vi "main.vi"() -> ()   [LabVIEW 2018]
doc: "This example demonstrates the use of binary morphological reconstruction in the particle analysis. The example allows you to keep the particles completely inside the ROI, completely outside the ROI or on the ROI."
uses:
  <vilib>/vision/NI_Vision_Development_Module.lvlib
panel:
  in  "Font, Size & Style":T1={"Desired Font (Application)"=enum."Application Font", "[User-specified Font]"={"Font Name"="", "Size"=12, "Strikeout?"=FALSE, "Italic?"=FALSE, "Underline?"=FALSE, "Outline?"=FALSE, "Shadow?"=FALSE, "Bold?"=FALSE, "Rotation Angle"=0.0}, "Horizontal Alignment"=0, "Vertical Alignment"=0} {"Horizontal Alignment" items=["Left", "Center", "Right"]; "Vertical Alignment" items=["Bottom", "Top", "Baseline"]}
  in  "Font, Size & Style 3":T1={"Desired Font (Application)"=enum."Application Font", "[User-specified Font]"={"Font Name"="", "Size"=12, "Strikeout?"=FALSE, "Italic?"=FALSE, "Underline?"=FALSE, "Outline?"=FALSE, "Shadow?"=FALSE, "Bold?"=FALSE, "Rotation Angle"=0.0}, "Horizontal Alignment"=0, "Vertical Alignment"=0} {"Vertical Alignment" items=["Bottom", "Top", "Baseline"]; "Horizontal Alignment" items=["Left", "Center", "Right"]; "[User-specified Font]"."Rotation Angle" format="%.2f"}
  out "总面积":i32
  out "ROI左上角坐标":cluster{i32, i32}
  out "透射图灰度表":u32[](graph)
  out "全图灰度级信息":T2 {"标准差" format="%.2f"; "均值" format="%.2f"; "相邻灰度级间隔" format="%.2f"; "起始灰度值" format="%.2f"; "最大值" format="%.2f"; "最小值" format="%.2f"}
  out "最大灰度值":sgl
  out "标注图":T3(plugin-control)
  out "写入数据库路径":path
  out "反射图灰度表":u32[](graph)
  out "反射图":T3(plugin-control)
  out "最大灰度值":sgl
  out "框数":dbl
  out "全图灰度级信息":T2 {"标准差" format="%.2f"; "均值" format="%.2f"; "相邻灰度级间隔" format="%.2f"; "起始灰度值" format="%.2f"; "最大值" format="%.2f"; "最小值" format="%.2f"}
  in  "评定报告生成":bool
  in  "部位":string
  in  "产品序号":string
  in  "测试人":string
  in  "预处理":bool
  in  "查看标注":bool
  in  "导入图像":bool
  in  "删除标注":bool
  in  "退出":bool
  in  "Font, Size & Style 2":T1={"Desired Font (Application)"=enum."Application Font", "[User-specified Font]"={"Font Name"="", "Size"=12, "Strikeout?"=FALSE, "Italic?"=FALSE, "Underline?"=FALSE, "Outline?"=FALSE, "Shadow?"=FALSE, "Bold?"=FALSE, "Rotation Angle"=0.0}, "Horizontal Alignment"=0, "Vertical Alignment"=0} {"Vertical Alignment" items=["Bottom", "Top", "Baseline"]; "Horizontal Alignment" items=["Left", "Center", "Right"]; "[User-specified Font]"."Rotation Angle" format="%.2f"}
  out "框组":T4(array[cluster])
  in  "Operation":enum16{"overlay rectangle"}(ring)
  # "穿透法图像"
  # "反射法图像"
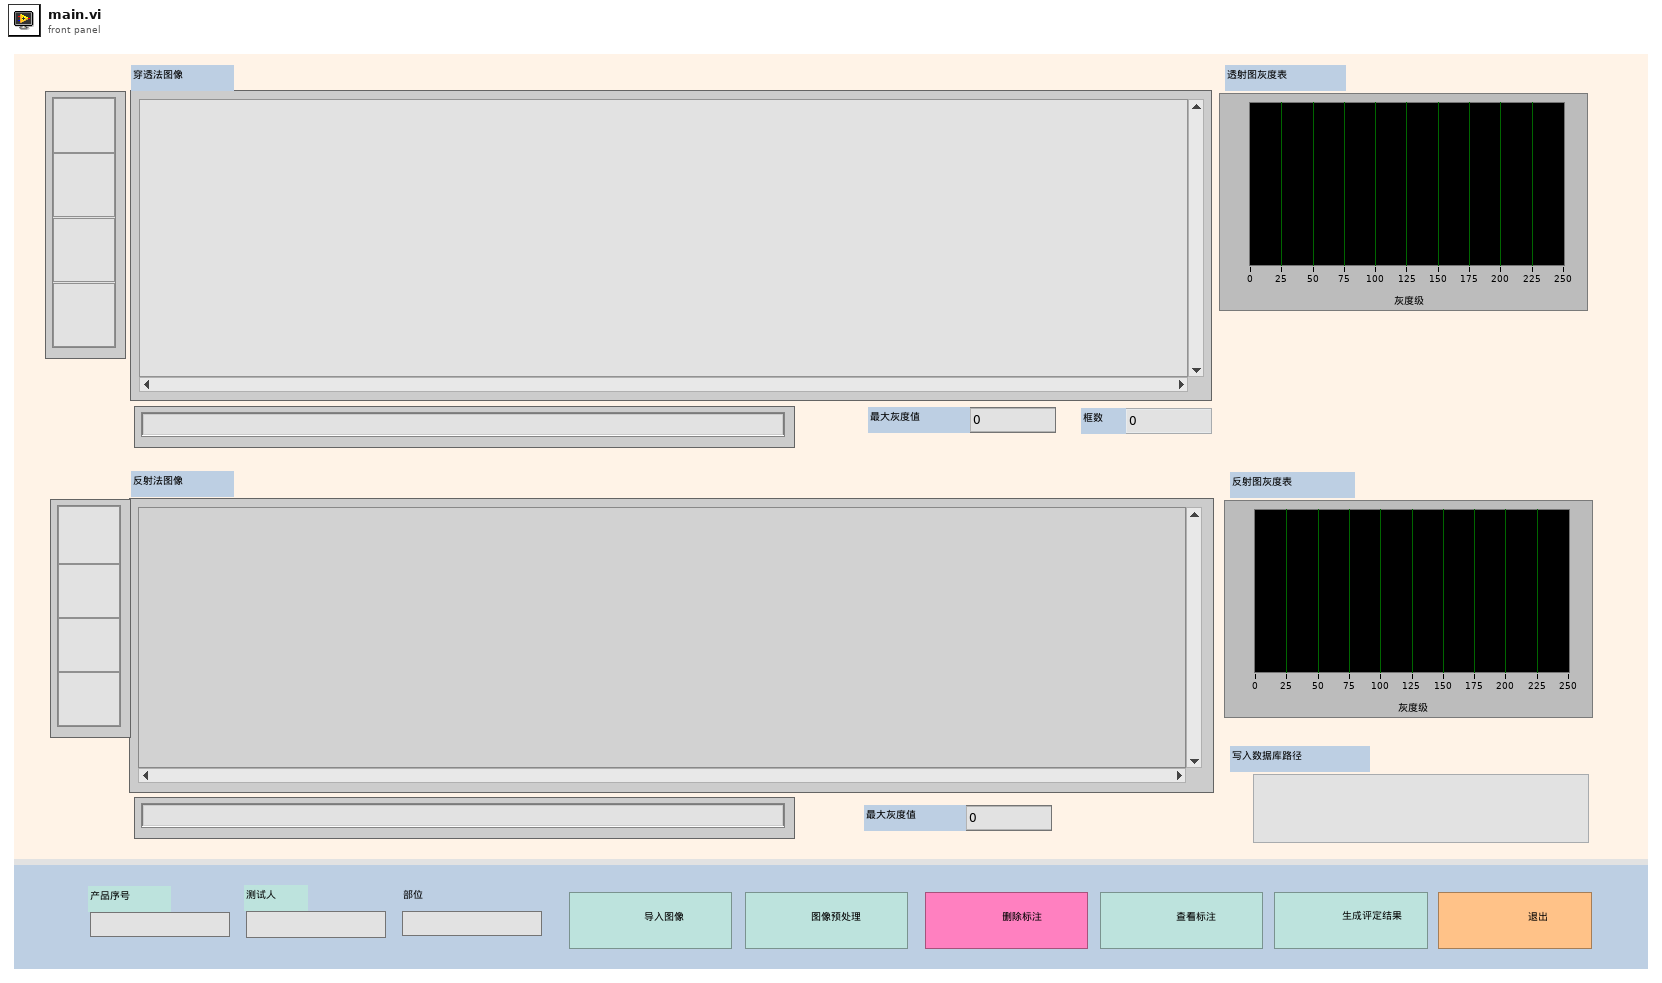
[diagram p1: front panel]
types:
  T1 = cluster{"Desired Font (Application)":enum16{"User-specified Font", "Application Font", "System Font", "Dialog Font"}, "[User-specified Font]":cluster{"Font Name":string, "Size":i16, "Strikeout?":bool, "Italic?":bool, "Underline?":bool, "Outline?":bool, "Shadow?":bool, "Bold?":bool, "Rotation Angle":dbl}, "Horizontal Alignment":i16, "Vertical Alignment":i16}
  T2 = cluster{"histogram":u32[], "最小值":sgl, "最大值":sgl, "起始灰度值":sgl, "相邻灰度级间隔":sgl, "均值":sgl, "标准差":sgl, "像素面积":i32}
  T3 = typedef "IMAQ Image.ctl" = refnum<image>
  T4 = cluster{"Global Rectangle":i32[], "Contours":cluster{"Contour Type":u32, "ROI Type":u32, "Points":i32[]}[]}[]
  T5 = typedef "Image Type" = u32
  T6 = cluster{"Global Rectangle":i32[], "Contours":cluster{"Contour Type":u32, "ROI Type":u32, "Points":i32[]}[]}
  T7 = cluster{"histogram":u32[], "Minimal Value":sgl, "Maximal Value":sgl, "Starting Value":sgl, "Interval Width":sgl, "Mean Value":sgl, "Standard  Variation":sgl, "Area (pixels)":i32}
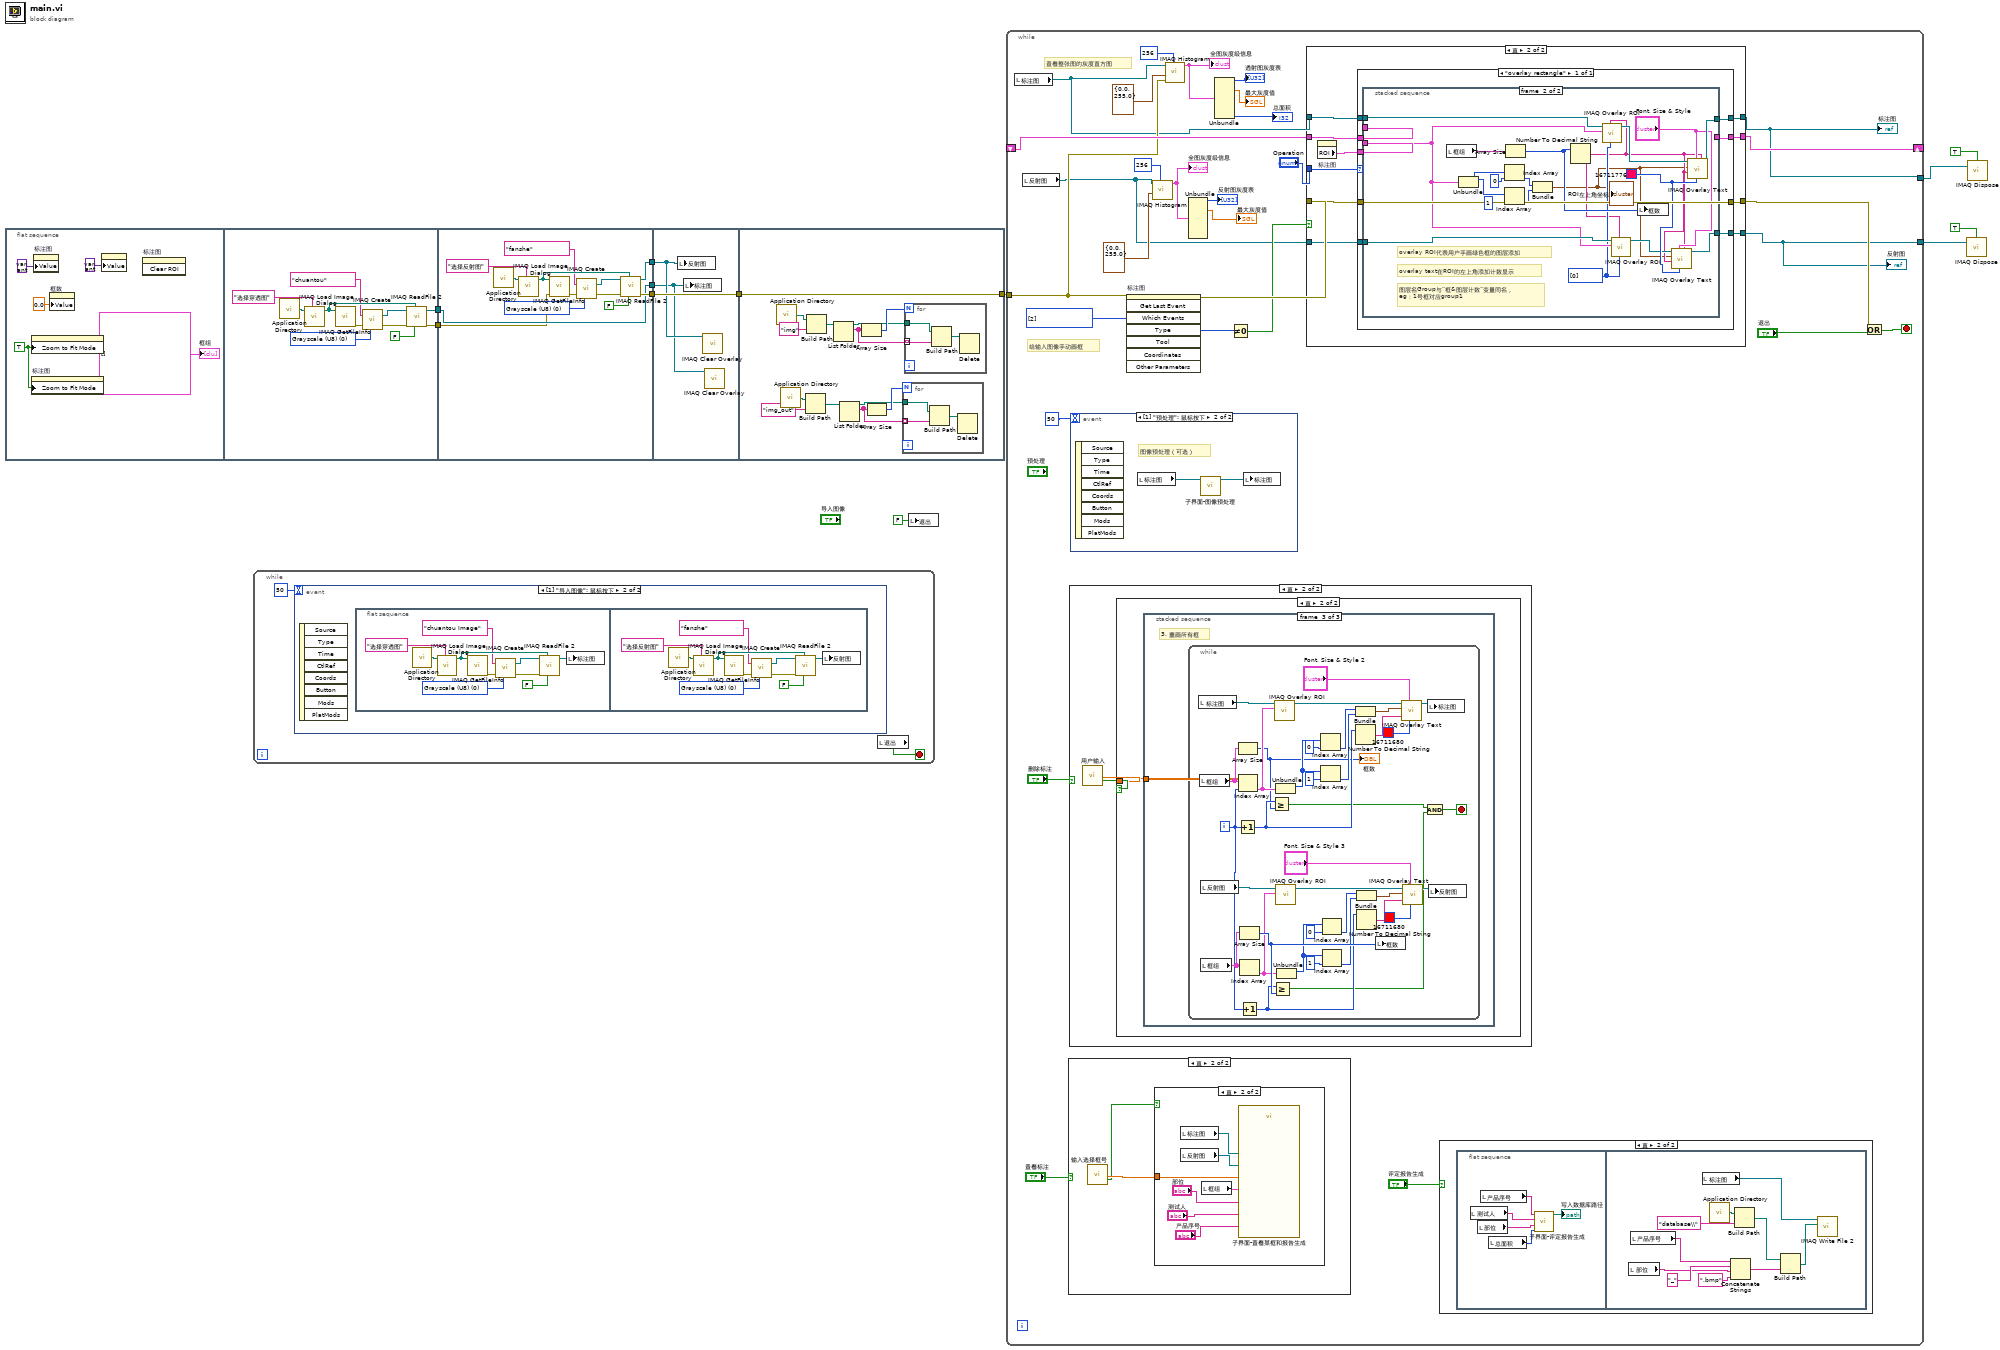
[diagram p0: block diagram]
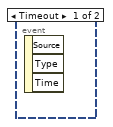
[diagram p2: hidden frame]
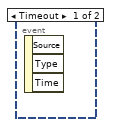
[diagram p4: hidden frame]
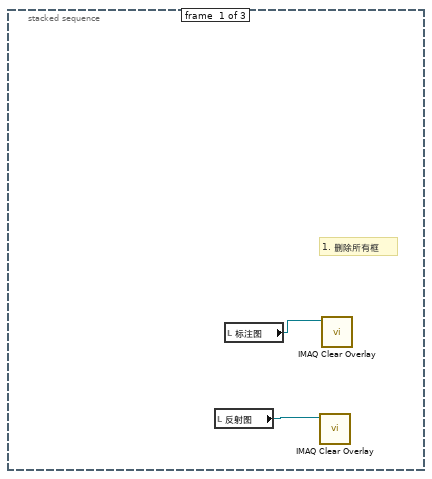
[diagram p9: hidden frame]
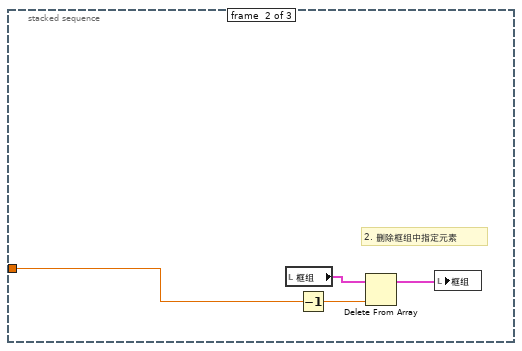
[diagram p10: hidden frame]
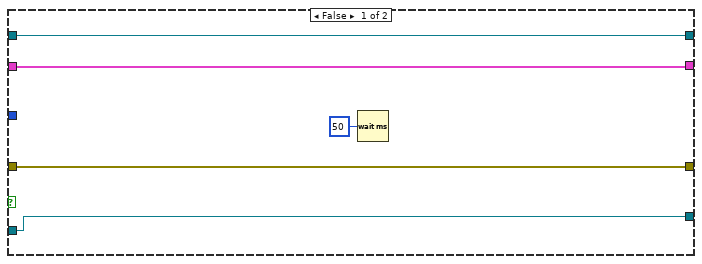
[diagram p11: hidden frame]
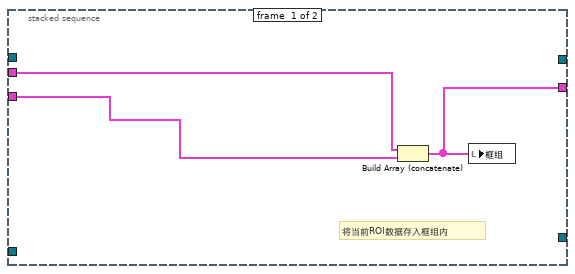
[diagram p12: hidden frame]
diagram:
  n1 = flat-sequence {
    tunnel: [w19] -> w9
    tunnel: [w18] -> w8
    tunnel: w9 -> [w30]
    tunnel: w8 -> [w31]
    tunnel: [w32] -> w7
    tunnel: [w31] -> w6
    tunnel: [w29] -> w5
    tunnel: w7 -> [w44]
    tunnel: w6 -> [w42]
    tunnel: w5 -> [w43]
    tunnel: [w44] -> w1
    tunnel: [w57] -> w12
    tunnel: w1 -> [w57]
    frame #0 {
      w16 = TRUE ("Zoom to Fit Mode")
      n2 = property on="反射图" class="ImageControl"("Zoom to Fit Mode"=w16) -> ()  [unwired: 2 in, 2 out]
      n3 = property on="标注图" class="ImageControl"("Zoom to Fit Mode"=w16) -> ()  [unwired: 2 in, 2 out]
      n4 = property on="标注图" class="ImageControl"("Value"=variant ("值")) -> ()  [unwired: 2 in, 2 out]
      n5 = property on="框数" class="DigNum (严格)"("Value"=0.0 ("标注框总数")) -> ()  [unwired: 2 in, 2 out]
      n6 = property on="反射图" class="ImageControl"("Value"=variant ("值")) -> ()  [unwired: 2 in, 2 out]
      n7 = invoke on="标注图" class="ImageControl" method="Clear ROI"() -> ()  [unwired: 3 in, 3 out]
      "框组" <- T4 [] ("框组")
    }
    frame #1 {
      w20 = T5 0 items=["Grayscale (U8)", "Grayscale (I16)", "Grayscale (SGL)", "Complex (CSG)", "RGB (U32)", "HSL (U32)", "RGB (U64)", "Grayscale (U16)"] ("Image Type")
      n8 = call <vilib>:"Application Directory.vi"() -> ("Application Directory"=w28:path)
      n9 = call "IMAQ Load Image Dialog"("Prompt"="选择穿透图" ("prompt"), "Start Path"=w28) -> ("Path"=w24:path)  [unwired: 7 in, 2 out]
      n10 = call "IMAQ GetFileInfo"("File Path"=w24) -> ("error out"=w25:errorcluster)  [unwired: 4 in, 6 out]
      n11 = call "IMAQ Create"("Image Name"="chuantou", "Image Type"=w20, "error in (no error)"=w25) -> ("New Image"=w26:T3, "error out"=w27:errorcluster)  [unwired: 2 in]
      n12 = call "IMAQ ReadFile 2"("Use File Path Image Type"=FALSE, "File Path"=w24, "error in (no error)"=w27, "Image"=w26) -> ("error out"=w19:errorcluster, "Image Out"=w18:T3)  [unwired: 3 in, 3 out]
    }
    frame #2 {
      w33 = T5 0 items=["Grayscale (U8)", "Grayscale (I16)", "Grayscale (SGL)", "Complex (CSG)", "RGB (U32)", "HSL (U32)", "RGB (U64)", "Grayscale (U16)"] ("Image Type")
      n13 = call <vilib>:"Application Directory.vi"() -> ("Application Directory"=w41:path)
      n14 = call "IMAQ Load Image Dialog"("Prompt"="选择反射图" ("prompt"), "Start Path"=w41) -> ("Path"=w37:path)  [unwired: 7 in, 2 out]
      n15 = call "IMAQ GetFileInfo"("error in (no error)"=w30, "File Path"=w37) -> ("error out"=w38:errorcluster)  [unwired: 3 in, 6 out]
      n16 = call "IMAQ Create"("Image Name"="fanshe", "Image Type"=w33, "error in (no error)"=w38) -> ("New Image"=w39:T3, "error out"=w40:errorcluster)  [unwired: 2 in]
      n17 = call "IMAQ ReadFile 2"("Use File Path Image Type"=FALSE, "File Path"=w37, "error in (no error)"=w40, "Image"=w39) -> ("error out"=w32:errorcluster, "Image Out"=w29:T3)  [unwired: 3 in, 3 out]
    }
    frame #3 {
      n18 = local write "反射图"(w43) -> ()
      n19 = local write "标注图"(w42) -> ()
      n20 = call "IMAQ Clear Overlay"("Image"=w43) -> ()  [unwired: 9 in, 2 out]
      n21 = call "IMAQ Clear Overlay"("Image"=w42) -> ()  [unwired: 9 in, 2 out]
    }
    frame #4 {
      n22 = call <vilib>:"Application Directory.vi"() -> ("Application Directory"=w53:path)
      n23 = call <vilib>:"Application Directory.vi"() -> ("Application Directory"=w47:path)
      n24 = Build Path(base path=w47, name or relative path="img_out" ("名称或相对路径")) -> (appended path=w48:path)
      n25 = Build Path(base path=w53, name or relative path="img" ("名称或相对路径")) -> (appended path=w54:path)
      n26 = List Folder(path=w54) -> (path out=w52:path, filenames=w56:string[])  [unwired: 3 in, 2 out]
      n27 = List Folder(path=w48) -> (path out=w46:path, filenames=w50:string[])  [unwired: 3 in, 2 out]
      n28 = Array Size(array=w56) -> (size(s)=w55:i32)
      n29 = Array Size(array=w50) -> (size(s)=w49:i32)
      n30 = for {
        N: w49 -> [_]
        tunnel: w46 -> [w59]
        tunnel: w50 -> [w58] mode=indexing
        n31 = Build Path(base path=w59, name or relative path=w58) -> (appended path=w60:path)
        n32 = Delete(path (use dialog)=w60) -> ()  [unwired: 4 in, 3 out]
      }
      n33 = for {
        N: w55 -> [_]
        tunnel: w52 -> [w62]
        tunnel: w56 -> [w61] mode=indexing
        n34 = Build Path(base path=w62, name or relative path=w61) -> (appended path=w63:path)
        n35 = Delete(path (use dialog)=w63) -> ()  [unwired: 4 in, 3 out]
      }
    }
  }
  n36 = while {
    stop <- w64 stop-if-true
    n37 = event shown="[1] \"导入图像\": 鼠标按下" {
      selector: _ -> [_ _]
      dyn-events: _ -> [_ _]
      timeout: 50 -> [_ _]
      event Timeout {
        n38 = event-data() -> ()  [unwired: 1 in, 3 out]
      }
      event "导入图像": Mouse Down {
        n39 = event-data() -> ()  [unwired: 1 in, 8 out]
        n40 = flat-sequence {
          frame #0 {
            w67 = T5 0 items=["Grayscale (U8)", "Grayscale (I16)", "Grayscale (SGL)", "Complex (CSG)", "RGB (U32)", "HSL (U32)", "RGB (U64)", "Grayscale (U16)"] ("Image Type")
            n41 = call <vilib>:"Application Directory.vi"() -> ("Application Directory"=w75:path)
            n42 = call "IMAQ Load Image Dialog"("Prompt"="选择穿透图" ("prompt"), "Start Path"=w75) -> ("Path"=w71:path)  [unwired: 7 in, 2 out]
            n43 = call "IMAQ GetFileInfo"("File Path"=w71) -> ("error out"=w72:errorcluster)  [unwired: 4 in, 6 out]
            n44 = call "IMAQ Create"("Image Name"="chuantou Image", "Image Type"=w67, "error in (no error)"=w72) -> ("New Image"=w73:T3, "error out"=w74:errorcluster)  [unwired: 2 in]
            n45 = call "IMAQ ReadFile 2"("Use File Path Image Type"=FALSE, "File Path"=w71, "error in (no error)"=w74, "Image"=w73) -> ("Image Out"=w66:T3)  [unwired: 3 in, 4 out]
            n46 = local write "标注图"(w66) -> ()
          }
          frame #1 {
            w79 = T5 0 items=["Grayscale (U8)", "Grayscale (I16)", "Grayscale (SGL)", "Complex (CSG)", "RGB (U32)", "HSL (U32)", "RGB (U64)", "Grayscale (U16)"] ("Image Type")
            n47 = call <vilib>:"Application Directory.vi"() -> ("Application Directory"=w81:path)
            n48 = call "IMAQ Load Image Dialog"("Prompt"="选择反射图" ("prompt"), "Start Path"=w81) -> ("Path"=w85:path)  [unwired: 7 in, 2 out]
            n49 = call "IMAQ GetFileInfo"("File Path"=w85) -> ("error out"=w84:errorcluster)  [unwired: 4 in, 6 out]
            n50 = call "IMAQ Create"("Image Name"="fanshe", "Image Type"=w79, "error in (no error)"=w84) -> ("New Image"=w83:T3, "error out"=w82:errorcluster)  [unwired: 2 in]
            n51 = call "IMAQ ReadFile 2"("Use File Path Image Type"=FALSE, "File Path"=w85, "error in (no error)"=w82, "Image"=w83) -> ("Image Out"=w76:T3)  [unwired: 3 in, 4 out]
            n52 = local write "反射图"(w76) -> ()
          }
        }
      }
    }
    n53 = local read "退出"() -> (w64:bool)
  }
  n54 = local write "退出"(FALSE ("退出")) -> ()
  n55 = while {
    shift-right: [w108] -> _
    shift-left: _ -> [w107]
    tunnel: w12 -> [w106]
    tunnel: [w90] -> w10
    tunnel: [w91] -> w3
    stop <- w110 stop-if-true
    (unwired) "_" ("名称或相对路径")
    (unwired) ".docx" ("名称或相对路径")
    w113 = i32[] [2] items=["No Event"=0, "Click Event"=1, "Draw Event"=2, "Size Event"=4, "Scroll Event"=5, "Double Click Event"=8] ("Which Events")
    # "给输入图像手动画框"
    # "查看整张图的灰度直方图"
    n56 = local read "标注图"() -> (w92:T3)
    n57 = local read "反射图"() -> (w93:T3)
    n58 = case shown="真" "查看标注" {
      frame False {
      }
      frame True {
        n59 = call "输入选择框号"() -> ("框号"=w134:dbl, "确定"=w133:bool)  [unwired: 17 in, 1 out]
        n60 = case shown="真" w133 {
          tunnel: w134 -> [_ w141]
          frame False {
            # "用户取消操作"
          }
          frame True {
            n61 = local read "标注图"() -> (w138:T3)
            n62 = local read "反射图"() -> (w139:T3)
            n63 = local read "框组"() -> (w140:T4)
            n64 = call "子界面-查看某框和报告生成.vi"("测试人"="测试人", "标注图"=w138, "部位"="部位", "产品序号"="产品序号", "反射图"=w139, "框组"=w140, "框号"=w141) -> ()  [unwired: 3 in]
          }
        }
      }
    }
    n65 = case shown="真" "删除标注" {
      frame False {
      }
      frame True {
        n66 = call "用户输入"() -> ("框号"=w142:dbl, "确定"=w143:bool)  [unwired: 17 in, 1 out]
        n67 = case shown="真" w143 {
          tunnel: w142 -> [_ w144]
          frame False {
            # "用户取消操作"
          }
          frame True {
            n68 = stacked-sequence {
              tunnel: w144 -> [_ w149 _]
              frame #0 {
                # "1. 删除所有框"
                n69 = local read "反射图"() -> (w145:T3)
                n70 = local read "标注图"() -> (w146:T3)
                n71 = call "IMAQ Clear Overlay"("Image"=w145) -> ()  [unwired: 9 in, 2 out]
                n72 = call "IMAQ Clear Overlay"("Image"=w146) -> ()  [unwired: 9 in, 2 out]
              }
              frame #1 {
                # "2. 删除框组中指定元素"
                n73 = local read "框组"() -> (w150:T4)
                n74 = Decrement(x=w149) -> (x-1=w148:dbl)
                n75 = Delete From Array(array=w150, index=w148) -> (array with subset deleted=w147:T4)  [unwired: 1 in, 1 out]
                n76 = local write "框组"(w147) -> ()
              }
              frame #2 {
                # "3. 重画所有框"
                n77 = while {
                  i -> [w155]
                  stop <- w152 stop-if-true
                  n78 = local read "标注图"() -> (w186:T3)
                  n79 = local read "框组"() -> (w180:T4)
                  n80 = local read "反射图"() -> (w156:T3)
                  n81 = local read "框组"() -> (w162:T4)
                  n82 = Array Size(array=w180) -> (size(s)=w171:i32)
                  "框数" <- w171
                  n83 = Index Array(array=w180, index=w155) -> (element=w173:T6)
                  n84 = Increment(x=w155) -> (x+1=w185:i32)
                  n85 = Array Size(array=w162) -> (size(s)=w170:i32)
                  n86 = Index Array(array=w162) -> (element=w169:T6)  [unwired: 1 in]
                  n87 = Increment(x=w155) -> (x+1=w157:i32)
                  n88 = Greater Or Equal?(x=w185, y=w171) -> (x >= y?=w154:bool)
                  n89 = Greater Or Equal?(x=w157, y=w170) -> (x >= y?=w153:bool)
                  n90 = call "IMAQ Overlay ROI"("ROI Descriptor"=w173, "Image"=w186) -> ("Image Out"=w182:T3)  [unwired: 8 in, 1 out]
                  n91 = Unbundle(w173) -> ("Global Rectangle"=w176:i32[])  [unwired: 1 out]
                  n92 = call "IMAQ Overlay ROI"("ROI Descriptor"=w169, "Image"=w156) -> ("Image Out"=w160:T3)  [unwired: 8 in, 1 out]
                  n93 = Unbundle(w169) -> ("Global Rectangle"=w166:i32[])  [unwired: 1 out]
                  n94 = Index Array(array=w176, index=0 ("索引")) -> (element=w177:i32)
                  n95 = Index Array(array=w176, index=1 ("索引")) -> (element=w178:i32)
                  n96 = Index Array(array=w166, index=0 ("索引")) -> (element=w165:i32)
                  n97 = Index Array(array=w166, index=1 ("索引")) -> (element=w164:i32)
                  n98 = Bundle(w177, w178) -> (w175:cluster{i32, i32})  [unwired: 1 in]
                  n99 = Number To Decimal String(number=w185) -> (decimal integer string=w183:string)  [unwired: 1 in]
                  n100 = Bundle(w165, w164) -> (w167:cluster{i32, i32})  [unwired: 1 in]
                  n101 = Number To Decimal String(number=w157) -> (decimal integer string=w159:string)  [unwired: 1 in]
                  n102 = local write "框数"(w170) -> ()
                  n103 = call "IMAQ Overlay Text"("Text Color (black)"=u32 16711680, "Font, Size & Style"="Font, Size & Style 2", "String"=w183, "Origin"=w175, "Image"=w182) -> ("Image Out"=w181:T3)  [unwired: 5 in, 1 out]
                  n104 = call "IMAQ Overlay Text"("Text Color (black)"=u32 16711680, "Font, Size & Style"="Font, Size & Style 3", "String"=w159, "Origin"=w167, "Image"=w160) -> ("Image Out"=w161:T3)  [unwired: 5 in, 1 out]
                  n105 = And(x=w154, y=w153) -> (x .and. y?=w152:bool)
                  n106 = local write "标注图"(w181) -> ()
                  n107 = local write "反射图"(w161) -> ()
                }
              }
            }
          }
        }
      }
    }
    n108 = event shown="[1] \"预处理\": 鼠标按下" {
      selector: _ -> [_ _]
      dyn-events: _ -> [_ _]
      timeout: 50 -> [_ _]
      event Timeout {
        n109 = event-data() -> ()  [unwired: 1 in, 3 out]
      }
      event "预处理": Mouse Down {
        # "图像预处理（可选）"
        n110 = event-data() -> ()  [unwired: 1 in, 8 out]
        n111 = local read "标注图"() -> (w132:T3)
        n112 = call "子界面-图像预处理.vi"("原图"=w132) -> ("处理后"=w131:T3)  [unwired: 10 in]
        n113 = local write "标注图"(w131) -> ()
      }
    }
    n114 = invoke on="标注图" class="ImageControl" method="Get Last Event"(error in=w106, "Which Events"=w113) -> (error out=w112:errorcluster, "Type"=w114:i32)  [unwired: 6 in, 6 out]
    n115 = call "IMAQ Histogram"("Number of Classes"=256, "Interval Range"=cluster{"Minimum":sgl, "Maximum":sgl} {"Minimum"=0.0, "Maximum"=255.0}, "Image"=w93) -> ("Histogram Report"=w95:T7)  [unwired: 7 in, 1 out]
    "全图灰度级信息" <- w95
    n116 = call "IMAQ Histogram"("Number of Classes"=256, "error in (no error)"=w106, "Interval Range"=cluster{"Minimum":sgl, "Maximum":sgl} {"Minimum"=0.0, "Maximum"=255.0}, "Image"=w92) -> ("Histogram Report"=w97:T7)  [unwired: 6 in, 1 out]
    "全图灰度级信息" <- w97
    n117 = Unbundle(w95) -> ("histogram"=→"反射图灰度表":u32[], "Maximal Value"=→"最大灰度值":sgl)  [unwired: 6 out]
    n118 = Unbundle(w97) -> ("histogram"=→"透射图灰度表":u32[], "Maximal Value"=→"最大灰度值":sgl, "Area (pixels)"=→"总面积":i32)  [unwired: 5 out]
    n119 = Not Equal To 0?(x=w114) -> (x != 0?=w109:bool)
    n120 = case shown="真" w109 {
      tunnel: w92 -> [w191 w201]
      tunnel: [w191 w200] -> w90
      tunnel: "Operation" -> [_ w198]
      tunnel: w112 -> [w190 w197]
      tunnel: [w190 w196] -> w111
      tunnel: [w188 w195] -> w108
      tunnel: w107 -> [w188 w194]
      tunnel: w93 -> [w187 w193]
      tunnel: [w187 w192] -> w91
      frame False {
        n121 = Wait (ms)(milliseconds to wait=u32 50) -> ()  [unwired: 1 out]
      }
      frame True {
        n122 = property on="标注图" class="ImageControl"() -> ("ROI"=w199:T6)  [unwired: 2 in, 2 out]
        n123 = case shown="\"overlay rectangle\"" w198 {
          tunnel: w201 -> [w208]
          tunnel: w199 -> [w206]
          tunnel: [w207] -> w200
          tunnel: w197 -> [w209]
          tunnel: [w209] -> w196
          tunnel: [w205] -> w195
          tunnel: w194 -> [w204]
          tunnel: w193 -> [w203]
          tunnel: [w202] -> w192
          frame "overlay rectangle" {
            n124 = stacked-sequence {
              tunnel: w208 -> [_ w224]
              tunnel: [_ w223] -> w207
              tunnel: w206 -> [w212 w220]
              tunnel: [w210 _] -> w205
              tunnel: w204 -> [w211 _]
              tunnel: w203 -> [_ w221]
              tunnel: [_ w217] -> w202
              frame #0 {
                # "将当前ROI数据存入框组内"
                n125 = Build Array (concatenate)(w211, w212) -> (w210:T4)
                n126 = local write "框组"(w210) -> ()
              }
              frame #1 {
                w215 = u32[] [0] ("Colors (Green)")
                w218 = u32 16711776 ("Text Color (black)")
                # "图层名Group与“框&图层计数”变量同名，\neg：1号框对应group1"
                # "overlay text在ROI的左上角添加计数显示"
                # "overlay ROI代表用户手画绿色框的图层添加"
                n127 = local read "框组"() -> (w227:T4)
                n128 = Unbundle(w220) -> ("Global Rectangle"=w230:i32[])  [unwired: 1 out]
                n129 = Index Array(array=w230, index=0 ("索引")) -> (element=w229:i32)
                n130 = Index Array(array=w230, index=1 ("索引")) -> (element=w228:i32)
                n131 = Array Size(array=w227) -> (size(s)=w222:i32)
                n132 = Bundle(w229, w228) -> (w213:cluster{i32, i32})  [unwired: 1 in]
                "ROI左上角坐标" <- w213
                n133 = Number To Decimal String(number=w222) -> (decimal integer string=w214:string)  [unwired: 1 in]
                n134 = call "IMAQ Overlay ROI"("Colors (Green)"=w215, "Group"=w214, "ROI Descriptor"=w220, "Image"=w224) -> ("Image Out"=w231:T3)  [unwired: 6 in, 1 out]
                n135 = call "IMAQ Overlay ROI"("Colors (Green)"=w215, "Group"=w214, "ROI Descriptor"=w220, "Image"=w221) -> ("Image Out"=w216:T3)  [unwired: 6 in, 1 out]
                n136 = local write "框数"(w222) -> ()
                n137 = call "IMAQ Overlay Text"("Group"=w214, "Text Color (black)"=w218, "Font, Size & Style"="Font, Size & Style", "String"=w214, "Origin"=w213, "Image"=w216) -> ("Image Out"=w217:T3)  [unwired: 4 in, 1 out]
                n138 = call "IMAQ Overlay Text"("Group"=w214, "Text Color (black)"=w218, "Font, Size & Style"="Font, Size & Style", "String"=w214, "Origin"=w213, "Image"=w231) -> ("Image Out"=w223:T3)  [unwired: 4 in, 1 out]
              }
            }
          }
        }
      }
    }
    "标注图" <- w90
    "反射图" <- w91
    n139 = case shown="真" "评定报告生成" {
      frame False {
      }
      frame True {
        n140 = flat-sequence {
          frame #0 {
            n141 = local read "测试人"() -> (w117:string)
            n142 = local read "部位"() -> (w118:string)
            n143 = local read "产品序号"() -> (w116:string)
            n144 = local read "总面积"() -> (w119:i32)
            n145 = call "子界面-评定报告生成.vi"("产品序号"=w116, "测试人"=w117, "部位"=w118, "总面积"=w119) -> ("写入数据库路径"=→"写入数据库路径":path)  [unwired: 6 in]
          }
          frame #1 {
            n146 = local read "部位"() -> (w124:string)
            n147 = local read "产品序号"() -> (w125:string)
            n148 = local read "标注图"() -> (w130:T3)
            n149 = call <vilib>:"Application Directory.vi"() -> ("Application Directory"=w123:path)
            n150 = Concatenate Strings(w125, "_" ("名称或相对路径"), w124, ".bmp" ("名称或相对路径")) -> (w129:string)
            n151 = Build Path(base path=w123, name or relative path="database\\" ("名称或相对路径")) -> (appended path=w121:path)
            n152 = Build Path(base path=w121, name or relative path=w129) -> (appended path=w126:path)
            n153 = call-poly "IMAQ Write File 2"("File Path"=w126, "Image"=w130) -> ()  [unwired: 8 in, 2 out]
          }
        }
      }
    }
    n154 = Or(x=w111, y="退出") -> (x .or. y?=w110:bool)
    n155 = call <vilib>:"Application Directory.vi"() -> ()  [unwired: 1 out]
  }
  n156 = call "IMAQ Dispose"("All Images? (No)"=TRUE, "Image"=w3) -> ()  [unwired: 1 in, 4 out]
  n157 = call "IMAQ Dispose"("All Images? (No)"=TRUE, "Image"=w10) -> ()  [unwired: 1 in, 4 out]
